vi "Execute Single SQL Statement.vi"(8 "error in (no error)":errorcluster, 10 "SQL statement":string caption="SQL (single statement)", 11 "SQLite Connection in":refnum<class "Connection.lvclass">) -> (0 "error out":errorcluster, 3 "SQLite Connection out":refnum<class "Connection.lvclass">)   [LabVIEW 2023, in "SQLiteSupport.lvlib" / "Connection.lvclass"]
doc: "Exectutes a single SQL statement (any additional statements are ignored)."
uses:
  Connection.lvclass
  SQL Statement/SQL Statement.lvclass
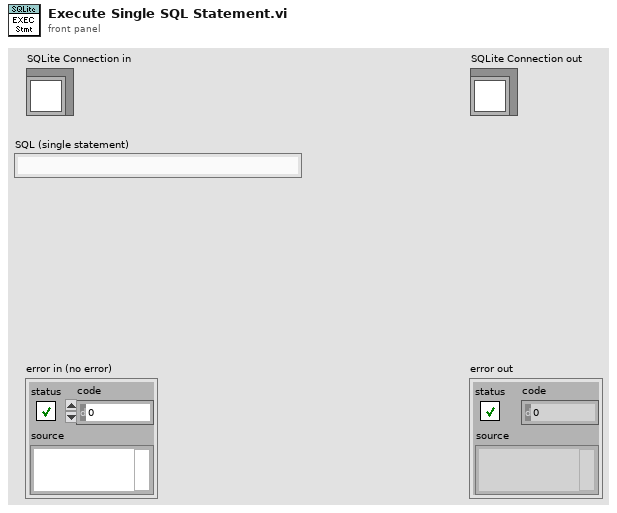
[diagram p1: front panel]
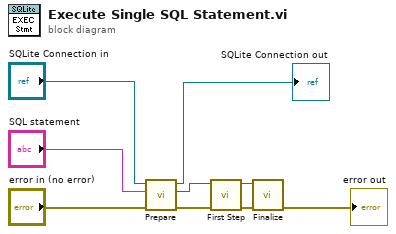
[diagram p0: block diagram]
diagram:
  n1 = call "Prepare.vi"("error in (no error)"="error in (no error)", "SQL"="SQL statement", "SQLite Connection in"="SQLite Connection in") -> ("error out"=w3:errorcluster, "SQL Statement out"=w5:refnum<class "SQL Statement.lvclass">, "SQLite Connection out"=→"SQLite Connection out":refnum<class "Connection.lvclass">)  [unwired: 4 in, 2 out]
  n2 = call "First Step.vi"("error in (no error)"=w3, "SQL Statement in"=w5) -> ("error out"=w2:errorcluster, "SQL Statement out"=w4:refnum<class "SQL Statement.lvclass">)  [unwired: 7 in, 1 out]
  n3 = call "Finalize.vi"("error in (no error)"=w2, "SQL Statement in"=w4) -> ("error out"=→"error out":errorcluster)  [unwired: 9 in]
